vi "Bridge Tipping Routine.vi"   [LabVIEW 2011]
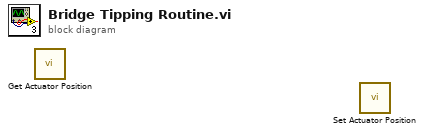
[diagram p0: block diagram]
diagram:
  n1 = call "Get Actuator Position.vi"() -> ()  [unwired: 1 out]
  n2 = call "Set Actuator Position.vi"() -> ()  [unwired: 1 in]
